vi "2B_Tech Serial Data Recording & DECADE 2.0_test.vi"() -> ()   [LabVIEW 2014]
uses:
  <vilib>/Instr/_visa.llb/VISA Set IO Buffer Mask.ctl
  <vilib>/Instr/_visa.llb/VISA Flush IO Buffer Mask.ctl
  <vilib>/Platform/TimedLoop/XDataNode/timing_clust.ctl
  <vilib>/Platform/TimedLoop/XDataNode/nitl_modes.ctl
  <vilib>/Platform/TimedLoop/XDataNode/wakeup.ctl
  C:/Program Files (x86)/National Instruments/LabVIEW 2014/examples/Data Communication/Network Streams/Simple Network Streams/support/Network Stream Command.ctl
  <vilib>/Utility/error.llb/whitespace.ctl
  <vilib>/Instr/_visa.llb/VISA Configure Serial Port (Instr).vi
  <vilib>/Utility/tcp.llb/UDP Multicast Write-Only Open.vi
  <vilib>/platform/TimedLoop/XDataNode/XDataNode.xnode
  <vilib>/Platform/TimedLoop/XDataNode/XDNodeRunTimeDep.lvlib
panel:
  out "Default file name":string
  out "error out":errorcluster
  out "Ambient/Cabin":bool
  out "Stop File Write":bool
  in  "timeout (10sec)":u32=3000
  in  "VISA resource name":refnum<visa-resource-name>="ASRL2::INSTR"
  in  "Simulate 3 av":dbl
  in  "Simulate\nConc":i32
  in  "Simulate\nconc":bool
  in  "3hr_alm_thresh":i32=80
  out "3hrAvg_Alarm":bool
  out "Inst_Alarm":bool
  in  "Inst_alm_thresh":i32=220
  out "Time":string
  in  "Clear Display\nErrors":bool
  out "Read Error Counter\nfrom process loop":u32
  out "CABOZO UDP_ASCII_Out":string
  out "Ozo_array":string[](array[string])
  out "3hr_ozo_avg":dbl
  out "q_size":i32
  out "Data Output":string[](array[string])
  out "UDP packet\nSend status":bool
  out "TWBOZO UDP_ASCII_Out":string
  out "UDP_Out_Error":errorcluster
  out "UDP_Pack_num":u32
  out "Flight Number":string
  out "Number of times \nRead time out":u32
  out "Data Loop count":i32
  out "2B_Serial_error out":errorcluster
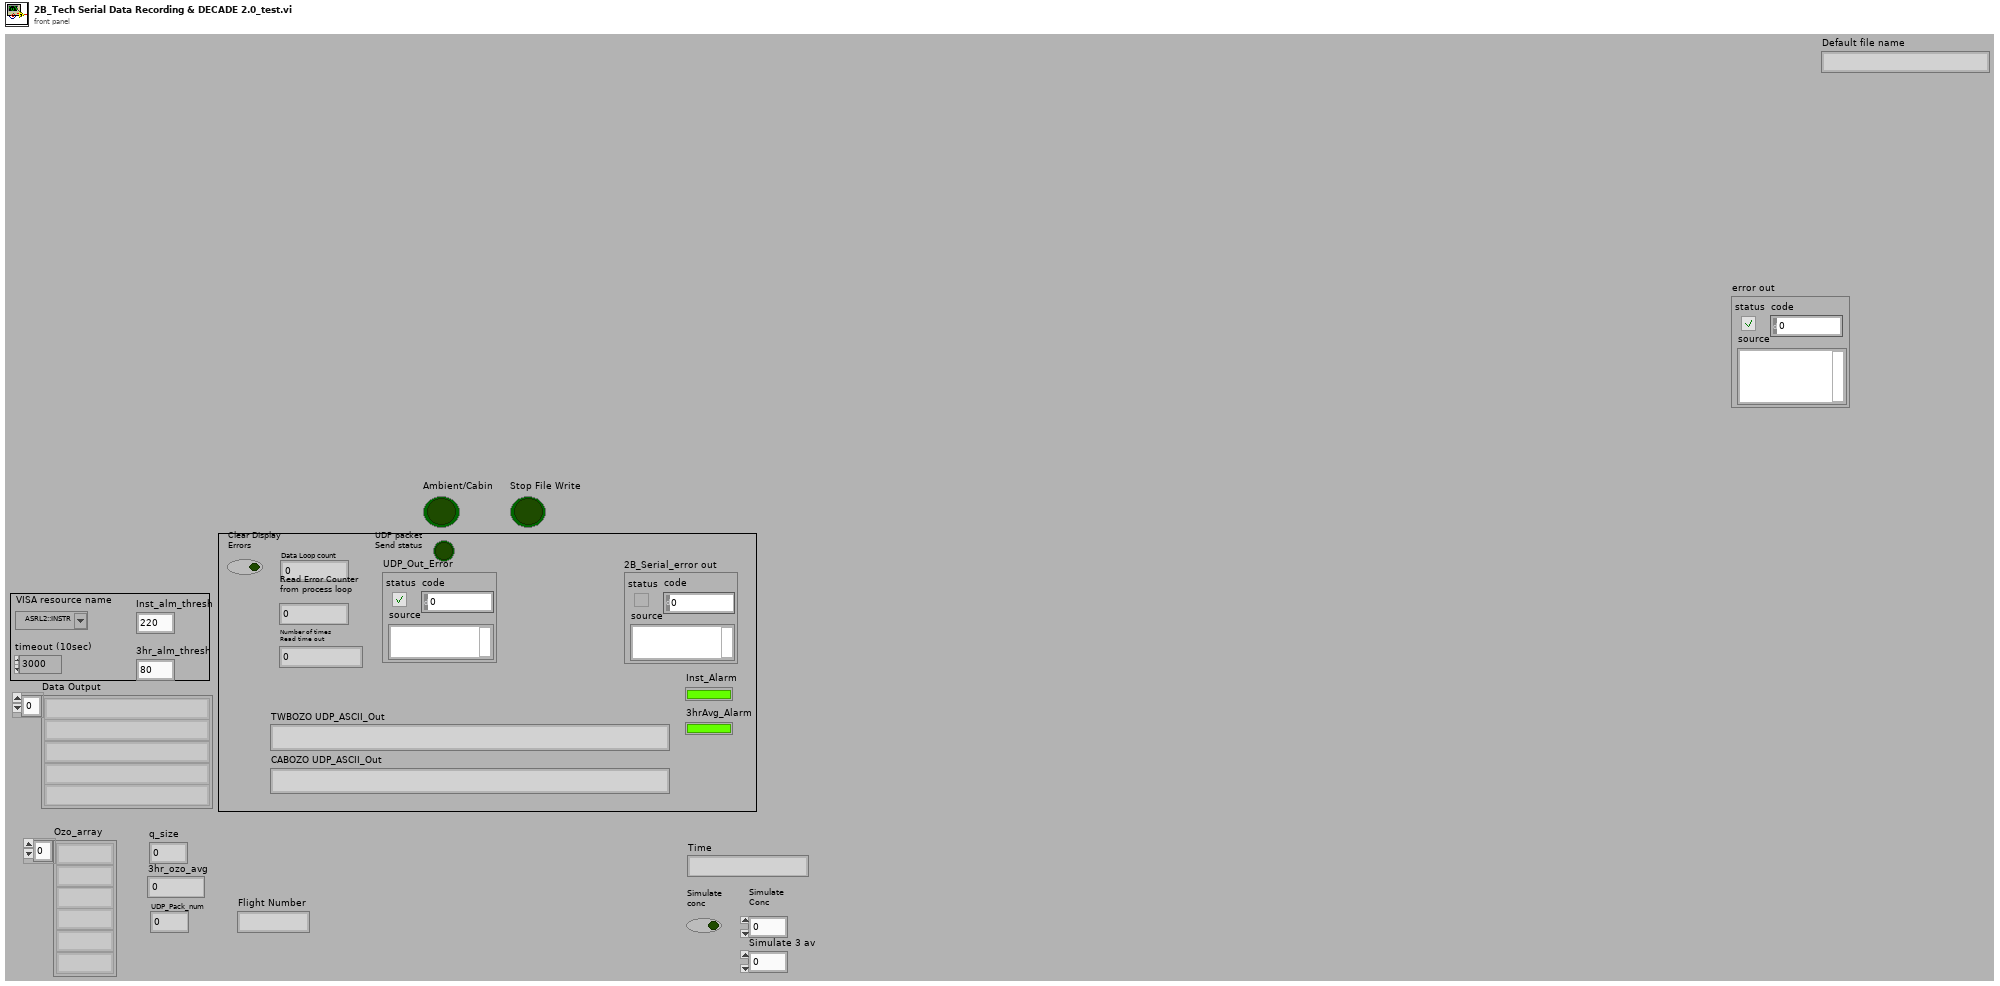
[diagram p1: front panel]
types:
  T1 = typedef "VISA Flush IO Buffer Mask.ctl" = u16
  T2 = typedef "VISA Set IO Buffer Mask.ctl" = u16
  T3 = typedef "Network Stream Command.ctl" = cluster{"Message":string, "Message Data":variant}
  T4 = typedef "XDNodeRunTimeDep.lvlib/timing_clust.ctl" = cluster{"Expected End [f-1]":u64, "Actual End [f-1]":u64, "Finished Late? [f-1]":bool, "Expected End [i-1]":u64, "Actual End [i-1]":u64, "Finished Late? [i-1]":bool, "Expected Start [i]":u64, "Actual Start [i]":u64, "Expected Start [f]":u64, "Actual Start [f]":u64, "Source Name":string, "Structure Name":string, "Period":i64, "Deadline":i64, "Offset":i64, "Start":i64, "Priority":i32, "Timeout":i32, "Mode":T5, "Wakeup Reason":T6, "Error":errorcluster, "Source Type":string, "Secondary Source Type":string, "Global End Time":u64, "Global Start Time":u64, "Frame Duration":u64, "Iteration Duration":u64, "Assigned CPU":i32, "I/O Scan Engine Mode":u32}
  T5 = typedef "XDNodeRunTimeDep.lvlib/nitl_modes.ctl" = enum32{"No Change", "Process missed periods, maintain original phase", "Discard missed periods, maintain original phase", "Process missed periods, ignore original phase", "Discard missed periods, ignore original phase"}
  T6 = typedef "XDNodeRunTimeDep.lvlib/wakeup.ctl" = enum32{"Normal", "Aborted", "Asynchronous wakeup", "Timing source error", "Timed loop error", "Timeout"}
  T7 = enum16{"open", "replace", "create", "open or create", "replace or create", "replace or create with confirmation"}
  T8 = typedef "whitespace.ctl" = u16
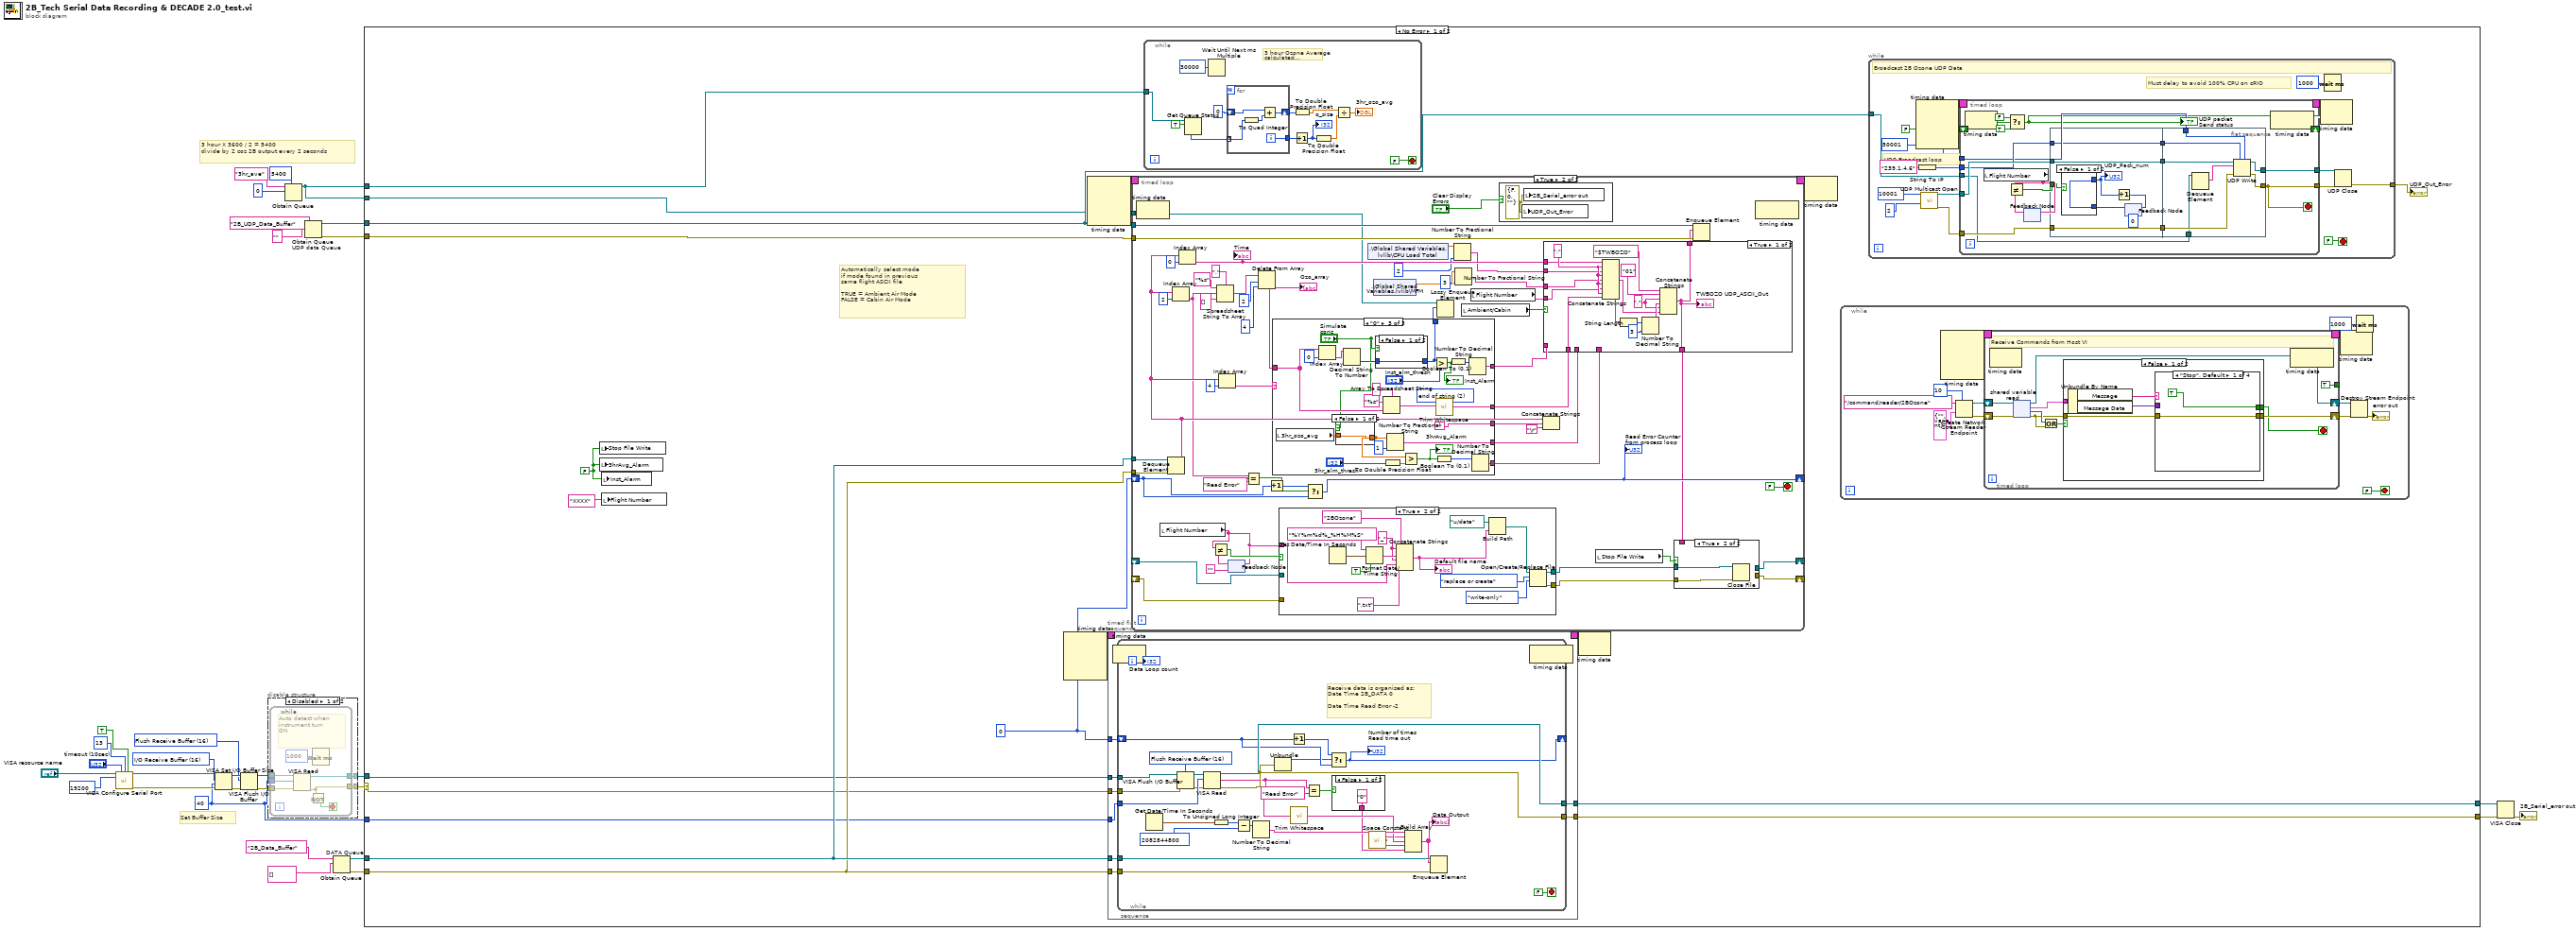
[diagram p0: block diagram]
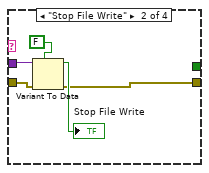
[diagram p3: hidden frame]
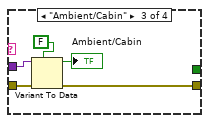
[diagram p4: hidden frame]
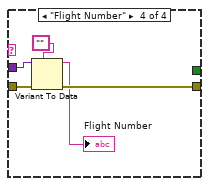
[diagram p5: hidden frame]
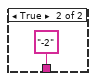
[diagram p7: hidden frame]
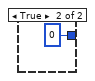
[diagram p8: hidden frame]
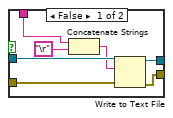
[diagram p9: hidden frame]
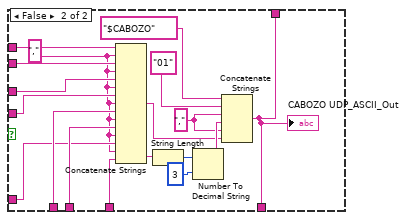
[diagram p12: hidden frame]
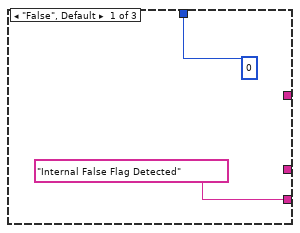
[diagram p13: hidden frame]
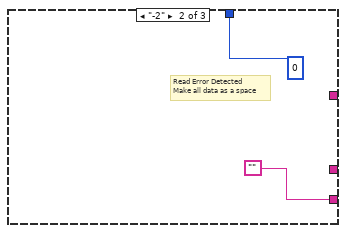
[diagram p14: hidden frame]
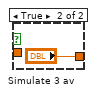
[diagram p15: hidden frame]
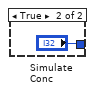
[diagram p16: hidden frame]
diagram:
  w1 = u32 40 ("size (4096)")
  w8 = T1 16 items=["Flush Receive Buffer"=16, "Write Transmit Buffer to Device"=32, "Flush Receive Buffer (No I/O)"=64, "Flush Transmit Buffer"=128] ("Mask")
  w9 = T2 16 items=["I/O Receive Buffer"=16, "I/O Transmit Buffer"=32, "I/O Receive and Transmit Buffer"=48] ("Mask")
  # "Set Buffer Size"
  # "3 hour X 3600 / 2 = 5400\ndivide by 2 coz 2B output every 2 seconds"
  n1 = call-poly "VISA Configure Serial Port"("VISA resource name"="VISA resource name", "timeout (10sec)"="timeout (10sec)", "termination char\n(0xA = '\\n' = LF)"=u8 13 ("termination char\n(0xA = '\\n' = LF)"), "Enable Termination\nChar (T)"=TRUE ("Enable Termination\nChar (T)"), "baud rate (9600)"=u32 19200) -> ("VISA resource name out"=w7:refnum<visa-resource-name>, "error out"=w6:errorcluster)  [unwired: 9 in]
  n2 = VISA Set I/O Buffer Size(VISA resource name=w7, mask (16)=w9, size (4096)=w1, error in (no error)=w6) -> (VISA resource name out=w10:refnum<visa-resource-name>, error out=w11:errorcluster)
  n3 = VISA Flush I/O Buffer(VISA resource name=w10, mask (16)=w8, error in (no error)=w11) -> (VISA resource name out=w5:refnum<visa-resource-name>, error out=w4:errorcluster)
  n4 = disable-structure shown="Disabled" {
    disable-tunnel: w5 -> [w36 _]
    disable-tunnel: w4 -> [w35 _]
    disable-tunnel: [w34 _] -> w3
    disable-tunnel: [w33 _] -> w2
    disable-tunnel: w1 -> [w32 _]
    frame Disabled {
      n5 = while {
        tunnel: w32 -> [w43]
        tunnel: w36 -> [w42]
        tunnel: w35 -> [w41]
        tunnel: [w39] -> w34
        tunnel: [w38] -> w33
        stop <- w40 stop-if-true
        # "Auto detect when\ninstrument turn\nON"
        n6 = VISA Read(VISA resource name=w42, byte count=w43, error in (no error)=w41) -> (VISA resource name out=w38:refnum<visa-resource-name>, error out=w39:errorcluster)  [unwired: 2 out]
        n7 = Not(x=w39) -> (.not. x?=w40:bool)
        n8 = Wait (ms)(milliseconds to wait=u32 1000) -> ()  [unwired: 1 out]
      }
    }
    frame Enabled {
    }
  }
  n9 = Obtain Queue(max queue size (-1, unlimited)=5400, name (unnamed)="3hr_ave", element data type=0 ("index")) -> (queue out=w17:refnum<queue>)  [unwired: 2 in, 2 out]
  n10 = Obtain Queue "UDP data Queue"(name (unnamed)="2B_UDP_Data_Buffer", element data type="") -> (queue out=w23:refnum<queue>, error out=w22:errorcluster)  [unwired: 3 in, 1 out]
  n11 = Obtain Queue "DATA Queue"(name (unnamed)="2B_Data_Buffer", element data type=string[] []) -> (queue out=w27:refnum<queue>, error out=w26:errorcluster)  [unwired: 3 in, 1 out]
  n12 = case shown="No Error" w3 {
    selector: w3 -> [w49 w385]
    tunnel: w2 -> [w50 w386]
    tunnel: [w62 w386] -> w30
    tunnel: [w54 w385] -> w31
    tunnel: w27 -> [w61 _]
    tunnel: w26 -> [w60 _]
    tunnel: w23 -> [w58 _]
    tunnel: w22 -> [w59 _]
    tunnel: w17 -> [w57 _]
    tunnel: w17 -> [w56 _]
    tunnel: w1 -> [w48 _]
    frame No Error {
      w45 = FALSE
      w55 = u32 0
      # "Automatically select mode\nif mode found in previous\nsame flight ASCII file\n\nTRUE = Ambient Air Mode\nFALSE = Cabin Air Mode"
      n13 = local write "Stop File Write"(w45) -> ()
      n14 = local write "3hrAvg_Alarm"(w45) -> ()
      n15 = local write "Inst_Alarm"(w45) -> ()
      n16 = local write "Flight Number"("XXXX" ("Flight Number")) -> ()
      n17 = node-c288() -> (w47:T4)  [unwired: 4 in]
      n18 = node-c288() -> (w53:T4)  [unwired: 4 in]
      n19 = timed-sequence {
        timing: w47 -> [_]
        timing-out: [_] -> w46
        tunnel: [w121] -> w62
        tunnel: w61 -> [w120]
        tunnel: w60 -> [w119]
        tunnel: w55 -> [w118]
        tunnel: [w117] -> w54
        tunnel: w50 -> [w116]
        tunnel: w49 -> [w115]
        tunnel: w48 -> [w114]
        n20 = timed-flat-sequence {
          tunnel: [w129] -> w121
          tunnel: w120 -> [w128]
          tunnel: w119 -> [w127]
          tunnel: w118 -> [w126]
          tunnel: [w125] -> w117
          tunnel: w116 -> [w124]
          tunnel: w115 -> [w123]
          tunnel: w114 -> [w122]
          n21 = node-c288() -> ()  [unwired: 1 in, 1 out]
          n22 = while {
            tunnel: [w148] -> w125
            shift-right: [w154] -> _
            shift-left: w126 -> [w155]
            tunnel: [w157] -> w129
            tunnel: w124 -> [w153]
            tunnel: w123 -> [w152]
            tunnel: w128 -> [w151]
            tunnel: w127 -> [w150]
            tunnel: w122 -> [w149]
            i -> [w156]
            stop <- FALSE stop-if-true
            w133 = T1 16 items=["Flush Receive Buffer"=16, "Write Transmit Buffer to Device"=32, "Flush Receive Buffer (No I/O)"=64, "Flush Transmit Buffer"=128] ("Mask")
            # "Receive data is organised as:\nDate Time 2B_DATA 0\n\nDate Time Read Error -2"
            n23 = Get Date/Time In Seconds() -> (seconds since 1Jan1904=w143:timestamp)
            n24 = VISA Flush I/O Buffer(VISA resource name=w153, mask (16)=w133, error in (no error)=w152) -> (VISA resource name out=w134:refnum<visa-resource-name>, error out=w132:errorcluster)
            n25 = VISA Read(VISA resource name=w134, byte count=w149, error in (no error)=w132) -> (VISA resource name out=w157:refnum<visa-resource-name>, read buffer=w131:string, error out=w148:errorcluster)  [unwired: 1 out]
            n26 = To Unsigned Long Integer(number=w143) -> (unsigned 32bit integer=w145:u32)
            n27 = Subtract(x=w145, y=u32 2082844800) -> (x-y=w142:u32)
            n28 = Number To Decimal String(number=w142) -> (decimal integer string=w139:string)  [unwired: 1 in]
            n29 = Unbundle(w148) -> ("status"=w146:bool)  [unwired: 2 out]
            n30 = Increment(x=w155) -> (x+1=w147:u32)
            n31 = call <vilib>:"Trim Whitespace.vi"("string"=w131) -> ("trimmed string"=w138:string)  [unwired: 1 in]
            n32 = Equal?(x=w131, y="Read Error") -> (x = y?=w140:bool)
            n33 = Select(t=w147, s=w146, f=w155) -> (s? t:f=w154:u32)
            "Number of times \nRead time out" <- w154
            n34 = case shown="False" w140 {
              tunnel: ["0" "-2"] -> w136
              frame False {
              }
              frame True {
              }
            }
            n35 = call <vilib>:"Space Constant.vi"() -> ("String"=w137:string)
            n36 = Build Array(w139, w137, w138, w137, w136) -> (w135:string[])
            "Data Output" <- w135
            n37 = Enqueue Element(queue=w151, element=w135, error in (no error)=w150) -> ()  [unwired: 1 in, 3 out]
            "Data Loop count" <- w156
          }
          n38 = node-c288() -> ()  [unwired: 1 in, 1 out]
        }
      }
      n39 = timed-loop {
        timing: w53 -> [_]
        timing-out: [_] -> w52
        tunnel: w61 -> [w289]
        tunnel: w60 -> [w288]
        tunnel: w58 -> [w287]
        tunnel: w59 -> [w286]
        tunnel: w56 -> [w258]
        shift-right: [w262] -> _
        shift-left: w55 -> [w263]
        shift-right: [w251] -> _
        shift-left: _ -> [w247]
        shift-right: [w245] -> _
        shift-left: _ -> [w246]
        stop <- FALSE stop-if-true
        n40 = node-c288() -> ()  [unwired: 1 in, 1 out]
        n41 = local read "Flight Number"() -> (w243:string)
        n42 = Dequeue Element(queue=w289, error in (no error)=w288) -> (element=w271:string[])  [unwired: 1 in, 3 out]
        n43 = Index Array(array=w271, index=2) -> (element=w264:string)
        n44 = Index Array(array=w271, index=0) -> (element=w273:string)
        "Time" <- w273
        n45 = Spreadsheet String To Array(delimiter (Tab)=",", format string="%s", spreadsheet string=w264, array type (2D Dbl)=string[] [] ("Values Array")) -> (array=w278:string[])
        n46 = Index Array(array=w271, index=4) -> (element=w279:string)
        n47 = feedback #1("" ("Flight Number")) -> (w253:string)
        n48 = Not Equal?(x=w243, y=w253) -> (x != y?=w244:bool)
        n49 = feedback-in #1(w243) -> ()
        n50 = Equal?(x=w264, y="Read Error") -> (x = y?=w266:bool)
        n51 = Delete From Array(array=w278, length=2, index=4) -> (array with subset deleted=w275:string[])  [unwired: 1 out]
        "Ozo_array" <- w275
        n52 = Increment(x=w263) -> (x+1=w265:u32)
        n53 = case shown="\"0\"" w279 {
          tunnel: w275 -> [_ _ w369]
          tunnel: [_ _ w372] -> w272
          tunnel: [0 0 w355] -> w257
          tunnel: ["Internal False Flag Detected" "" ""] -> w270
          tunnel: [_ _ w366] -> w268
          tunnel: [_ _ w362] -> w260
          tunnel: [_ _ w357] -> w259
          frame "False", Default {
          }
          frame "-2" {
            # "Read Error Detected\nMake all data as a space"
          }
          frame "0" {
            w373 = T8 2 items=["both", "start of string", "end of string"] ("location (both)")
            n54 = local read "3hr_ozo_avg"() -> (w353:dbl)
            n55 = Index Array(array=w369, index=0) -> (element=w370:string)
            n56 = case shown="False" "Simulate\nconc" {
              tunnel: [w377 "Simulate 3 av"] -> w352
              tunnel: w353 -> [w377 _]
              frame False {
              }
              frame True {
              }
            }
            n57 = Decimal String To Number(string=w370) -> (number=w356:i32)  [unwired: 2 in, 1 out]
            n58 = case shown="False" "Simulate\nconc" {
              tunnel: [w379 "Simulate\nConc"] -> w355
              tunnel: w356 -> [w379 _]
              frame False {
              }
              frame True {
              }
            }
            n59 = Array To Spreadsheet String(delimiter (Tab)=",", array=w369, 3:"%s" ("format string")) -> (spreadsheet string=w374:string)
            n60 = To Double Precision Float(number="3hr_alm_thresh") -> (double precision float=w359:dbl)
            n61 = Number To Fractional String(number=w352, precision (6)=i16 1) -> (F-format string=w366:string)  [unwired: 2 in]
            n62 = Greater?(x=w352, y=w359) -> (0:w360:bool)
            "3hrAvg_Alarm" <- w360
            n63 = Greater?(x=w355, y="Inst_alm_thresh") -> (0:w363:bool)
            "Inst_Alarm" <- w363
            n64 = call <vilib>:"Trim Whitespace.vi"("string"=w374, "location (both)"=w373) -> ("trimmed string"=w372:string)
            n65 = Boolean To (0,1)(Boolean=w360) -> (0, 1=w361:i16)
            n66 = Boolean To (0,1)(Boolean=w363) -> (0, 1=w364:i16)
            n67 = Number To Decimal String(number=w364) -> (decimal integer string=w362:string)  [unwired: 1 in]
            n68 = Number To Decimal String(number=w361) -> (decimal integer string=w357:string)  [unwired: 1 in]
          }
        }
        n69 = case shown="True" w244 {
          tunnel: [w300 w303] -> w249
          tunnel: [w299 w302] -> w248
          tunnel: w247 -> [w300 _]
          tunnel: w246 -> [w299 _]
          tunnel: w243 -> [_ w301]
          frame False {
          }
          frame True {
            w310 = "_" ("string")
            n70 = Get Date/Time In Seconds() -> (seconds since 1Jan1904=w311:timestamp)
            n71 = Format Date/Time String(time format string (%c)="%Y%m%d%_%H%M%S", seconds (now)=w311, UTC format=TRUE) -> (date/time string=w314:string)
            n72 = Concatenate Strings("2BOzone" ("string"), w310, w314, w310, w301, ".txt" ("string")) -> (w308:string)
            "Default file name" <- w308
            n73 = Build Path(base path=path "u:/data", name or relative path=w308) -> (appended path=w304:path)
            n74 = Open/Create/Replace File(file path (use dialog)=w304, operation (0:open)=T7."replace or create", access (0:read/write)=enum16{"read/write", "read-only", "write-only"}."write-only") -> (refnum out=w303:refnum<file>, error out=w302:errorcluster)  [unwired: 3 in, 1 out]
          }
        }
        n75 = Select(t=w265, s=w266, f=w263) -> (s? t:f=w262:u32)
        "Read Error Counter\nfrom process loop" <- w262
        n76 = shared-variable ".\\Global Shared Variables.lvlib\\CPU Load Total"() -> (w241:dbl)  [unwired: 1 in, 1 out]
        n77 = shared-variable ".\\Global Shared Variables.lvlib\\MFM"() -> (w239:dbl)  [unwired: 1 in, 1 out]
        n78 = Lossy Enqueue Element(queue=w258, element=w257) -> ()  [unwired: 1 in, 4 out]
        n79 = Number To Fractional String(number=w241, precision (6)=i16 2) -> (F-format string=w240:string)  [unwired: 2 in]
        n80 = Number To Fractional String(number=w239, precision (6)=i16 3) -> (F-format string=w236:string)  [unwired: 2 in]
        n81 = local read "Ambient/Cabin"() -> (w254:bool)
        n82 = local read "Flight Number"() -> (w255:string)
        n83 = case shown="True" "Clear Display\nErrors" {
          frame False {
          }
          frame True {
            w316 = errorcluster {"status"=FALSE, "code"=0, "source"=""} ("UDP Error Out")
            n84 = local write "UDP_Out_Error"(w316) -> ()
            n85 = local write "2B_Serial_error out"(w316) -> ()
          }
        }
        n86 = Concatenate Strings(w271, w270, "\r") -> ()  [unwired: 1 out]
        n87 = case shown="True" w254 {
          tunnel: [w317 w331] -> w285
          tunnel: w273 -> [w322 w340]
          tunnel: w272 -> [w321 w339]
          tunnel: w240 -> [w320 w338]
          tunnel: w236 -> [w319 w337]
          tunnel: w255 -> [w318 w336]
          tunnel: w268 -> [_ w335]
          tunnel: w260 -> [_ w334]
          tunnel: w259 -> [_ w332]
          tunnel: [w317 w331] -> w242
          frame True {
            w330 = ","
            w326 = ","
            n88 = Concatenate Strings(w322, w330, w320, w330, w319, w330, w318, w330, w321) -> (w325:string)
            n89 = String Length(string=w325) -> (length=w329:i32)
            n90 = Number To Decimal String(number=w329, width (-)=i16 3) -> (decimal integer string=w327:string)
            n91 = Concatenate Strings("$TWBOZO", "01", w326, w327, w326, w325) -> (w317:string)
            "TWBOZO UDP_ASCII_Out" <- w317
          }
          frame False {
            w333 = ","
            w344 = ","
            n92 = Concatenate Strings(w340, w333, w338, w333, w337, w333, w336, w333, w339, w333, w335, w333, w334, w333, w332) -> (w343:string)
            n93 = String Length(string=w343) -> (length=w347:i32)
            n94 = Number To Decimal String(number=w347, width (-)=i16 3) -> (decimal integer string=w345:string)
            n95 = Concatenate Strings("$CABOZO", "01", w344, w345, w344, w343) -> (w331:string)
            "CABOZO UDP_ASCII_Out" <- w331
          }
        }
        n96 = local read "Stop File Write"() -> (w250:bool)
        n97 = case shown="True" w250 {
          tunnel: w249 -> [w296 w298]
          tunnel: w248 -> [w295 w297]
          tunnel: [w292 _] -> w251
          tunnel: [w291 _] -> w245
          tunnel: w242 -> [w290 _]
          frame False {
            n98 = Concatenate Strings(w290, "\r") -> (w293:string)
            n99 = Write to Text File(file (use dialog)=w296, text=w293, error in=w295) -> (refnum out=w292:refnum<file>, error out=w291:errorcluster)  [unwired: 2 out]
          }
          frame True {
            n100 = Close File(refnum=w298, error in=w297) -> ()  [unwired: 2 out]
          }
        }
        n101 = Enqueue Element(queue=w287, element=w285, error in (no error)=w286) -> ()  [unwired: 1 in, 3 out]
        n102 = node-c288() -> ()  [unwired: 1 in, 1 out]
      }
      n103 = while {
        tunnel: w57 -> [w168]
        stop <- FALSE stop-if-true
        # "3 hour Ozone Average calculated\nevery 30 seconds"
        n104 = Get Queue Status(queue=w168, return elements? (F)=TRUE) -> (elements=w165:i32[])  [unwired: 1 in, 7 out]
        n105 = Wait Until Next ms Multiple(millisecond multiple=u32 30000) -> ()  [unwired: 1 out]
        n106 = for {
          tunnel: [w180] -> w175
          shift-right: [w179] -> w173
          shift-left: i64 0 -> [w178]
          tunnel: w165 -> [w176] mode=indexing
          i -> [w180]
          n107 = To Quad Integer(1:w176) -> (0:w177:i64)
          n108 = Add(x=w178, y=w177) -> (x+y=w179:i64)
        }
        n109 = Increment(x=w175) -> (x+1=w169:i32)
        "q_size" <- w169
        n110 = To Double Precision Float(number=w173) -> (double precision float=w171:dbl)
        n111 = To Double Precision Float(number=w169) -> (double precision float=w172:dbl)
        n112 = Divide(x=w171, y=w172) -> (x/y=→"3hr_ozo_avg":dbl)
      }
      n113 = node-c288(w46) -> ()  [unwired: 1 out]
      n114 = node-c288(w52) -> ()  [unwired: 1 out]
      n115 = while {
        stop <- FALSE stop-if-true
        n116 = node-c288() -> (w64:T4)  [unwired: 4 in]
        n117 = Create Network Stream Reader Endpoint(7:10 ("reader buffer size"), 9:T3 {"Message"="", "Message Data"=variant} ("Message Cluster"), 11:"/command/reader/2BOzone" ("reader url")) -> (0:w70:errorcluster, 3:w71:refnum<k21>)  [unwired: 4 in]
        n118 = timed-loop "Host->Target Command Reader" {
          shift-right: [w81] -> w68
          shift-left: w70 -> [w84]
          shift-right: [w82] -> w67
          shift-left: w71 -> [w83]
          tunnel: [TRUE] -> _
          timing: w64 -> [_]
          timing-out: [_] -> w63
          stop <- w75 stop-if-true
          # "Receive Commands from Host VI"
          n119 = node-c288() -> ()  [unwired: 1 in, 1 out]
          n120 = shared-variable-read(w83, w84) -> (w82:refnum<k21>, w77:errorcluster, w79:bool, w80:T3)  [unwired: 1 in]
          n121 = Or(x=w79, y=w77) -> (x .or. y?=w78:bool)
          n122 = case shown="False" w78 {
            selector: w78 -> [_ w110]
            tunnel: w77 -> [w92 w111]
            tunnel: [w91 w111] -> w81
            tunnel: w80 -> [w89 _]
            tunnel: [w90 w110] -> w75
            frame False {
              n123 = Unbundle By Name(w89) -> ("Message"=w88:string, "Message Data"=w87:variant)
              n124 = case shown="\"Stop\", Default" w88 {
                tunnel: w92 -> [w94 w99 w104 w109]
                tunnel: [w94 w95 w103 w108] -> w91
                tunnel: w87 -> [_ w98 w102 w107]
                tunnel: [TRUE _ _ _] -> w90
                frame "Stop", Default {
                }
                frame "Stop File Write" {
                  n125 = Variant To Data(error in=w99, type=FALSE, Variant=w98) -> (data=→"Stop File Write":bool, error out=w95:errorcluster)
                }
                frame "Ambient/Cabin" {
                  n126 = Variant To Data(error in=w104, type=FALSE, Variant=w102) -> (data=→"Ambient/Cabin":bool, error out=w103:errorcluster)
                }
                frame "Flight Number" {
                  n127 = Variant To Data(error in=w109, type="", Variant=w107) -> (data=→"Flight Number":string, error out=w108:errorcluster)
                }
              }
            }
            frame True {
            }
          }
          n128 = node-c288() -> ()  [unwired: 1 in, 1 out]
        }
        n129 = node-c288(w63) -> ()  [unwired: 1 out]
        n130 = Destroy Stream Endpoint(8:w68, 11:w67) -> (0:→"error out":errorcluster)
        n131 = Wait (ms)(milliseconds to wait=u32 1000) -> ()  [unwired: 1 out]
      }
      n132 = while {
        tunnel: w58 -> [w184]
        tunnel: [w183] -> w51
        stop <- FALSE stop-if-true
        # "Must delay to avoid 100% CPU on cRIO"
        # "UDP Broadcast loop"
        # "Broadcast 2B Ozone UDP Data"
        n133 = node-c288() -> (w186:T4)  [unwired: 4 in]
        n134 = String To IP(1:"239.1.4.6" ("name")) -> (0:w188:u32)
        n135 = call-poly <vilib>:"UDP Multicast Open.vi"("time-to-live (1)"=u16 2, "port"=u16 10001) -> ("error out"=w195:errorcluster, "connection ID"=w196:refnum<k16>)  [unwired: 8 in]
        n136 = timed-loop {
          tunnel: w196 -> [w213]
          tunnel: w195 -> [w212]
          tunnel: [w201] -> w191
          shift-right: [w198] -> _
          shift-left: FALSE -> [w206]
          tunnel: [w197] -> w190
          tunnel: w188 -> [w203]
          tunnel: u16 50001 ("port or service name") -> [w202]
          timing: w186 -> [_]
          timing-out: [_] -> w185
          tunnel: w184 -> [w199]
          stop <- w197 stop-if-true
          n137 = node-c288() -> ()  [unwired: 1 in, 1 out]
          n138 = local read "Flight Number"() -> (w200:string)
          n139 = Select(t=FALSE, s=w206, f=TRUE) -> (s? t:f=w198:bool)
          "UDP packet\nSend status" <- w198
          n140 = feedback-in #2(w200) -> ()
          n141 = feedback #2() -> (w208:string)  [unwired: 1 in]
          n142 = Not Equal?(x=w200, y=w208) -> (x != y?=w207:bool)
          n143 = flat-sequence {
            tunnel: w203 -> [w221]
            tunnel: w212 -> [w222]
            tunnel: w213 -> [w223]
            tunnel: [w223] -> w211
            tunnel: [w222] -> w210
            tunnel: [w221] -> w209
            tunnel: w207 -> [w220]
            tunnel: w202 -> [w233]
            tunnel: w211 -> [w232]
            tunnel: w210 -> [w231]
            tunnel: w209 -> [w230]
            tunnel: [w229] -> w201
            tunnel: [w228] -> w197
            tunnel: w199 -> [w226]
            frame #0 {
              n144 = feedback #3(u32 0) -> (w217:u32)
              n145 = case shown="False" w220 {
                tunnel: w217 -> [w224 _]
                tunnel: [w224 u32 0] -> w216
                frame False {
                }
                frame True {
                }
              }
              "UDP_Pack_num" <- w216
              n146 = Increment(x=w216) -> (x+1=w218:u32)
              n147 = feedback-in #3(w218) -> ()
            }
            frame #1 {
              n148 = Dequeue Element(queue=w226) -> (element=w227:string)  [unwired: 2 in, 3 out]
              n149 = UDP Write(address=w230, port or service name=w233, connection ID=w232, data in=w227, 8:w231) -> (error out=w228:errorcluster, 3:w229:refnum<k16>)  [unwired: 1 in]
            }
          }
          n150 = node-c288() -> ()  [unwired: 1 in, 1 out]
        }
        n151 = node-c288(w185) -> ()  [unwired: 1 out]
        n152 = Wait (ms)(milliseconds to wait=u32 1000) -> ()  [unwired: 1 out]
        n153 = UDP Close(connection ID=w191, 8:w190) -> (error out=w183:errorcluster)  [unwired: 1 out]
      }
      "UDP_Out_Error" <- w51
    }
    frame Error {
    }
  }
  n154 = VISA Close(VISA resource name=w30, error in (no error)=w31) -> (error out=→"2B_Serial_error out":errorcluster)
